vi "ifr2025 RF Offset.vi"(8 "error in (no error)":errorcluster {"code" format="%.0x"}, 9 "Offset (Enable)":bool=TRUE, 10 "Level (0.0)":dbl, 11 "instrument handle":refnum<visa-resource-name>) -> (0 "error out":errorcluster {"code" format="%.0x"}, 3 "instrument handle out":refnum<visa-resource-name>)   [LabVIEW 2009]
doc: "This VI specifies an RF output offset to compensate for cable or switching offsets. An offset is allowed for each output carrier frequency band."
uses:
  Ifr2025_32.dll
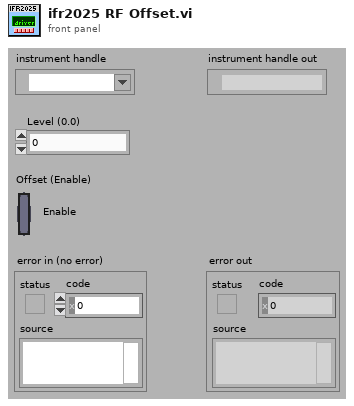
[diagram p1: front panel]
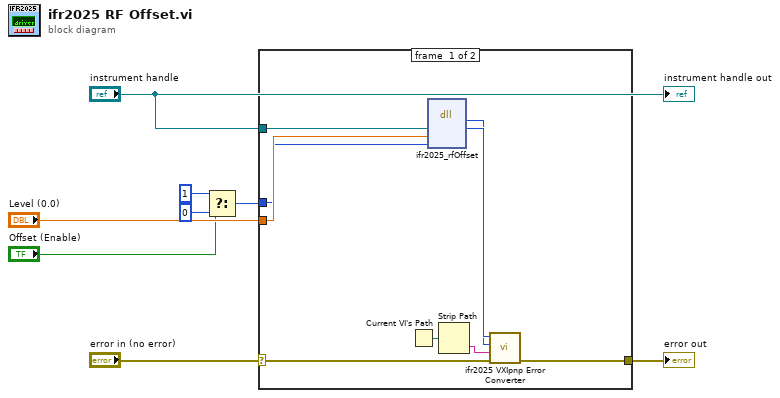
[diagram p0: block diagram]
diagram:
  n1 = Select(t=i16 1, s="Offset (Enable)", f=i16 0) -> (s? t:f=w1:i16)
  n2 = case shown="No Error" "error in (no error)" {
    selector: "error in (no error)" -> [w12 w18]
    tunnel: [w11 w18] -> w8
    tunnel: "instrument handle" -> [w16 _]
    tunnel: "Level (0.0)" -> [w10 _]
    tunnel: w1 -> [w9 _]
    frame #0 {
      n3 = Current VI's Path() -> (path=w17:path)
      n4 = dll-call lib="P:/inst/Marconi 2024 Signal Generator/source/labview/ifr2025/ifr2025/ifr2025_*.*" fn="ifr2025_rfOffset"("vi"=w16, "Level"=w10, "Offset"=w9) -> (w14:i32, "vi"=w15:u32)  [unwired: 5 in, 2 out]
      n5 = Strip Path(path=w17) -> (name=w13:string)  [unwired: 1 out]
      n6 = call "ifr2025 VXIpnp Error Converter.vi"("error in (no error)"=w12, "name of VI (\"\")"=w13, "CVI error code (0)"=w14, "instrument handle"=w15) -> ("error out"=w11:errorcluster)  [unwired: 7 out]
    }
    frame #1 {
    }
  }
  "error out" <- w8
  "instrument handle out" <- "instrument handle"
